vi "MT Generate Synchronization Parameters.vi"   [LabVIEW 2020, in "niDMT.lvlib"]
doc: "Constructs an FSK, PSK, QAM, MSK, PAM, ASK, or CPM <B>synchronization parameters</B> cluster that you can pass to a demodulation VI, using an array of either synchronization bits or synchronization numbers. The generated <B>synchronization parameters</B> cluster avoids phase ambiguity at the demodulator, thus allowing recovery of the actual message bits."
uses:
  <vilib>/addons/Modulation/niDMT.lvlib
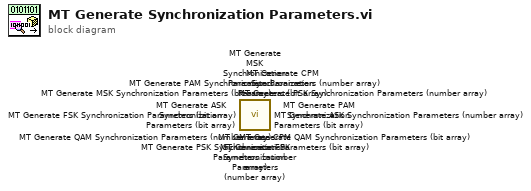
[diagram p0: block diagram]
diagram:
  n1 = call <vilib>:"MT Generate CPM Synchronization Parameters (number array).vi"() -> ()  [unwired: 14 in, 2 out]
  n2 = call <vilib>:"MT Generate CPM Synchronization Parameters (bit array).vi"() -> ()  [unwired: 14 in, 2 out]
  n3 = call <vilib>:"MT Generate ASK Synchronization Parameters (bit array).vi"() -> ()  [unwired: 14 in, 2 out]
  n4 = call <vilib>:"MT Generate PAM Synchronization Parameters (bit array).vi"() -> ()  [unwired: 14 in, 2 out]
  n5 = call <vilib>:"MT Generate MSK Synchronization Parameters (bit array).vi"() -> ()  [unwired: 14 in, 2 out]
  n6 = call <vilib>:"MT Generate QAM Synchronization Parameters (bit array).vi"() -> ()  [unwired: 14 in, 2 out]
  n7 = call <vilib>:"MT Generate PSK Synchronization Parameters (bit array).vi"() -> ()  [unwired: 14 in, 2 out]
  n8 = call <vilib>:"MT Generate FSK Synchronization Parameters (bit array).vi"() -> ()  [unwired: 14 in, 2 out]
  n9 = call <vilib>:"MT Generate ASK Synchronization Parameters (number array).vi"() -> ()  [unwired: 14 in, 2 out]
  n10 = call <vilib>:"MT Generate PAM Synchronization Parameters (number array).vi"() -> ()  [unwired: 14 in, 2 out]
  n11 = call <vilib>:"MT Generate QAM Synchronization Parameters (number array).vi"() -> ()  [unwired: 14 in, 2 out]
  n12 = call <vilib>:"MT Generate PSK Synchronization Parameters (number array).vi"() -> ()  [unwired: 14 in, 2 out]
  n13 = call <vilib>:"MT Generate MSK Synchronization Parameters (number array).vi"() -> ()  [unwired: 14 in, 2 out]
  n14 = call <vilib>:"MT Generate FSK Synchronization Parameters (number array).vi"() -> ()  [unwired: 14 in, 2 out]
